vi "Reset Computation.vi"(8 "error in (no error)":errorcluster, 11 "VISA resource name":refnum<visa-resource-name>) -> (0 "error out":errorcluster, 3 "VISA resource name out":refnum<visa-resource-name>)   [LabVIEW 2020, in "Yokogawa GX Series.lvlib"]
doc: "Resets computation."
uses:
  <instrlib>/Yokogawa GX Series/Yokogawa GX Series.lvlib
panel:
  in  "Batch Group Number  (0: OFF)":i32(ring) items=["OFF", "1", "2", "3", "4", "5", "6", "7", "8", "9", "10", "11", "12", "ALL"]
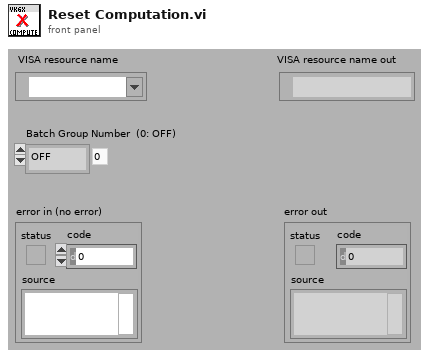
[diagram p1: front panel]
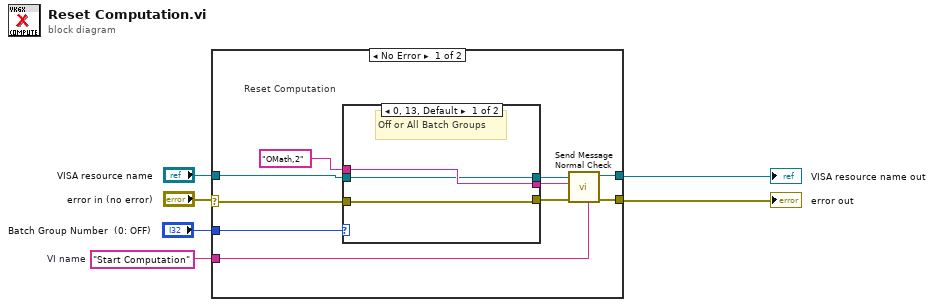
[diagram p0: block diagram]
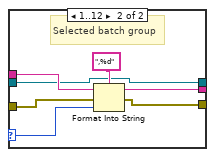
[diagram p2: hidden frame]
diagram:
  w3 = "Start Computation"  # VI name
  n1 = case shown="No Error" "error in (no error)" {
    selector: "error in (no error)" -> [w11 w27]
    tunnel: "VISA resource name" -> [w9 w28]
    tunnel: [w16 w28] -> w5
    tunnel: [w15 w27] -> w4
    tunnel: w3 -> [w14 _]
    tunnel: "Batch Group Number  (0: OFF)" -> [w7 _]
    frame No Error {
      # "Reset Computation"
      n2 = case shown="0, 13, Default" w7 {
        selector: w7 -> [_ w25]
        tunnel: "OMath,2" -> [w19 w24]
        tunnel: [w19 w23] -> w12
        tunnel: w11 -> [w18 w22]
        tunnel: [w18 w21] -> w10
        tunnel: w9 -> [w17 w20]
        tunnel: [w17 w20] -> w8
        frame 0, 13, Default {
          # "Off or All Batch Groups"
        }
        frame 1..12 {
          # "Selected batch group"
          n3 = Format Into String(format string=",%d", initial string=w24, error in=w22, w25) -> (resulting string=w23:string, error out=w21:errorcluster)
        }
      }
      n4 = call <instrlib>:"Send Message Normal Check.vi"("Source (\"\")"=w14, "error in (no error)"=w10, "Send Message (\"\")"=w12, "VISA resource name"=w8) -> ("error out"=w15:errorcluster, "VISA resource name out"=w16:refnum<visa-resource-name>)  [unwired: 2 in, 4 out]
    }
    frame Error {
    }
  }
  "error out" <- w4
  "VISA resource name out" <- w5
